vi "FindRequiredComponents.vi"(7 "Item Types (visible only)":T3 items=["all visible", "all including hidden", "standard only", "startup only"], 8 "error in (no error)":errorcluster, 9 "Component Version":string, 10 "Component ID":string, 11 "Session in":refnum<k21>) -> (0 "error out":errorcluster, 2 "Required Components":T1[](array[typedef]) {"Visibility Type" items=["standard", "hidden", "system", "unknown", "startup", "image"]}, 3 "Session out":refnum<k21>)   [LabVIEW 2014, in "nisyscfg.lvlib"]
uses:
  nisyscfg.lvlib
  Component Types.ctl
  Software Extended.ctl
  Component Type.ctl
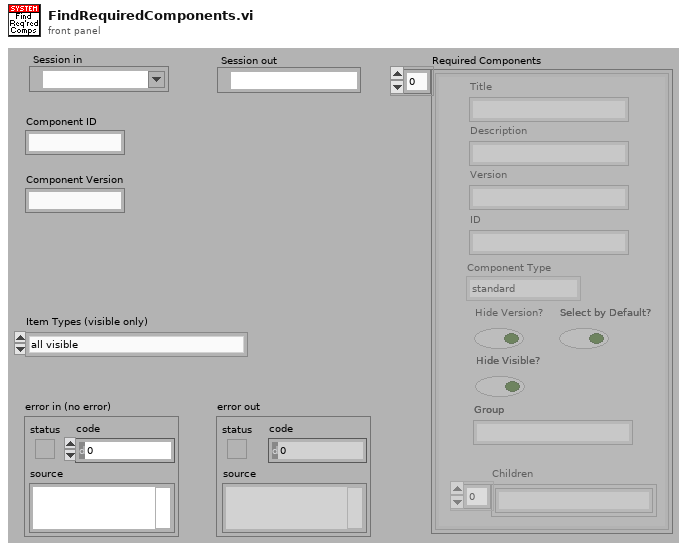
[diagram p1: front panel]
types:
  T1 = typedef "nisyscfg.lvlib/Software Extended.ctl" = cluster{"Description":string, "ID":string, "Version":string, "Title":string, "Visibility Type":T2, "Hide Version?":bool, "Children":string[], "Select by Default?":bool, "Hide Visible?":bool, "Group":string}
  T2 = typedef "nisyscfg.lvlib/Component Type.ctl" = u32
  T3 = typedef "nisyscfg.lvlib/Component Types.ctl" = u32
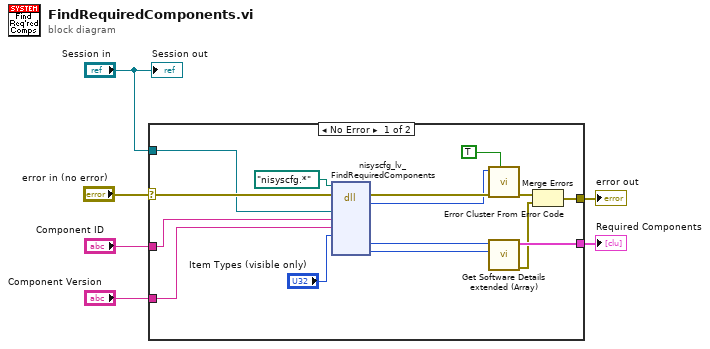
[diagram p0: block diagram]
diagram:
  n1 = case shown="No Error" "error in (no error)" {
    selector: "error in (no error)" -> [w19 w22]
    tunnel: "Session in" -> [w18 _]
    tunnel: "Component Version" -> [w16 _]
    tunnel: "Component ID" -> [w15 _]
    tunnel: [w9 w22] -> w2
    tunnel: [w13 _] -> w1
    frame No Error {
      n2 = dll-call lib="nisyscfg.*" fn="nisyscfg_lv_FindRequiredComponents" label="FindRequiredComponents"(path in=path "nisyscfg.*", error in=w19, "session"=w18, "componentID"=w15, "componentVersion"=w16, "includeTypes"="Item Types (visible only)") -> (error out=w21:errorcluster, "result"=w20:i32, "requiredComponents"=w12:u64, "numComponents"=w8:i32)  [unwired: 7 in, 1 out]
      n3 = call "Error Cluster From Error Code.vi"("show call chain? (False)"=TRUE, "error in (no error)"=w21, "error code (0)"=w20) -> ("error out"=w11:errorcluster)  [unwired: 6 in]
      n4 = call "Get Software Details extended (Array).vi"("Number of Elements"=w8, "Enumerator in"=w12) -> ("error out"=w10:errorcluster, "Software Components"=w13:T1[])  [unwired: 8 in]
      n5 = Merge Errors(w11, w10) -> (w9:errorcluster)
    }
    frame Error {
    }
  }
  "error out" <- w2
  "Required Components" <- w1
  "Session out" <- "Session in"
